vi "getIntegerValueList.vi"(8 "error in (no error)":errorcluster, 11 "IDict in":refnum<class "IDict.lvclass">) -> (0 "error out":errorcluster, 2 "Integer Value list out":i32[](array[numeric]), 3 "IDict out":refnum<class "IDict.lvclass">)   [LabVIEW 2022 SP3, in "openDAQ.lvlib" / "daqCoreTypes.lvlib" / "IDict.lvclass"]
uses:
  <instrlib>/openDAQ/Public/Classes/daqCoreTypes/IDict/IDict.lvclass
  C:/Program Files (x86)/National Instruments/LabVIEW 2022/instr.lib/openDAQ/Public/Classes/IBaseObject/IBaseObject.lvclass
  <instrlib>/openDAQ/Public/Classes/daqCoreTypes/IList/IList.lvclass
  <instrlib>/openDAQ/Public/Classes/IBaseObject/IBaseObject.lvclass/IBaseObject.ctl
  <instrlib>/openDAQ/Public/Classes/IBaseObject/Accessor/Read reference.vi
  <instrlib>/openDAQ/Public/Classes/IBaseObject/Accessor/Write reference.vi
  <instrlib>/openDAQ/Public/Classes/daqCoreTypes/IList/Polymorphic/getList/getIntegerList.vi
  <instrlib>/openDAQ/Binaries/Windows/x86/copendaq32.dll
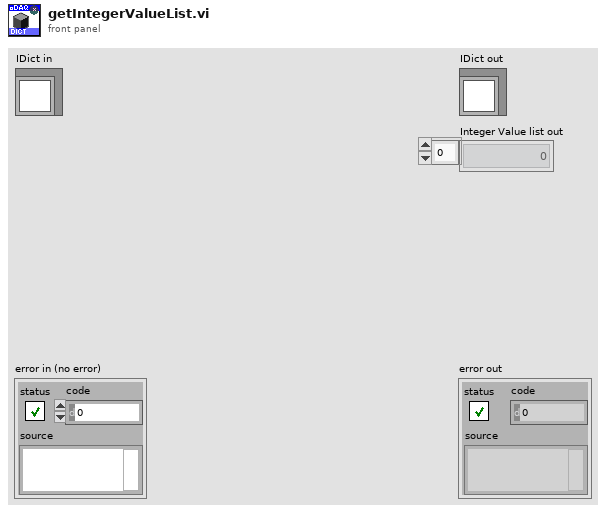
[diagram p1: front panel]
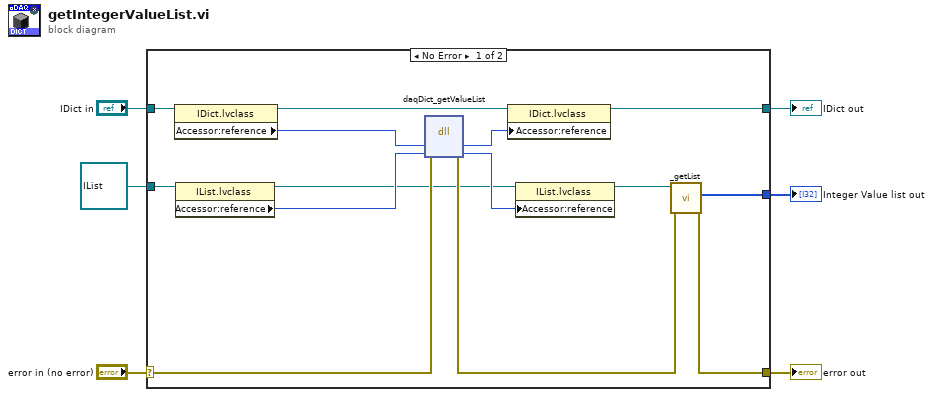
[diagram p0: block diagram]
diagram:
  n1 = case shown="No Error" "error in (no error)" {
    selector: "error in (no error)" -> [w17 w22]
    tunnel: [w8 w22] -> w5
    tunnel: [w13 w21] -> w3
    tunnel: "IDict in" -> [w16 w21]
    tunnel: refnum<class "IList.lvclass"> refnum ("openDAQ.lvlib:daqCoreTypes.lvlib:IList.lvclass") -> [w10 _]
    tunnel: [w7 _] -> w1
    frame No Error {
      n2 = property class="IDict.lvclass"(reference=w16) -> (reference out=w14:refnum<class "IDict.lvclass">, "Accessor:reference"=w15:i64)  [unwired: 1 in, 1 out]
      n3 = property class="IList.lvclass"(reference=w10) -> (reference out=w12:refnum<class "IList.lvclass">, "Accessor:reference"=w18:i64)  [unwired: 1 in, 1 out]
      n4 = dll-call lib="C:/Program Files (x86)/National Instruments/LabVIEW 2022/instr.lib/openDAQ/Binaries/Windows/x86/copendaq*.*" fn="daqDict_getValueList"(error in=w17, "dict"=w15, "valueList"=w18) -> (error out=w20:errorcluster, "dict"=w11:i64, "valueList"=w19:i64)  [unwired: 3 in, 1 out]
      n5 = property class="IDict.lvclass"(reference=w14, "Accessor:reference"=w11) -> (reference out=w13:refnum<class "IDict.lvclass">)  [unwired: 1 in, 1 out]
      n6 = property class="IList.lvclass"(reference=w12, "Accessor:reference"=w19) -> (reference out=w9:refnum<class "IList.lvclass">)  [unwired: 1 in, 1 out]
      n7 = call-poly <instrlib>:"_getList.vi"("error in (no error)"=w20, "IList in"=w9) -> ("error out"=w8:errorcluster, "Integers out"=w7:i32[])  [unwired: 8 in]
    }
    frame Error {
    }
  }
  "error out" <- w5
  "IDict out" <- w3
  "Integer Value list out" <- w1
